vi "Stop_Loop_Case.vi"(6 "Queues":T4, 7 "Timer parameters":refnum<vi>, 8 "Status/Errors in":refnum<vi>, 9 "Control Parameters [] in":T1[](array[typedef]) {"Aux Byte Value" format="%02x"; "Max Real Value" format="%#_6e"; "Min Real Value" format="%#_6e"; "dReal/dByte" format="%#_6e"; "Byte Value" format="%02x"; "Identifier" format="%02x"}, 10 "Main parameters in":T5={"Mode"={"Mode"=enum."Dialog", "Expert?"=FALSE, "Dialog?"=FALSE}, "Stop loop"={"Settings changed?"=FALSE, "Stop?"=refnum}, "Send message"={"Send mode"=enum."Get parameters", "Set parameter list"=0, "Get parameter list"=0, "Reset device"=0, "Length set settings message"=0, "Reset buttons?"=FALSE, "Reset Master?"=enum."General"}, "Write settings"={"Options"=enum."File 1"}, "Settings state"={"MAS locked?"=refnum, "SLV locked?"=refnum}, "Button refs"={"Stop program"=refnum, "Save settings"=refnum, "DAQ mode"=refnum, "Reset settings"=refnum, "Apply settings"=refnum, "Reset MAS"=refnum, "Reset SLV"=refnum, "Local DBase?"=refnum, "Last value DBase"=FALSE, "Database"=refnum, "Calibration"=refnum, "Save settings 2"=refnum}, "Update screen"={"Detector number"=0, "Hardware"=enum."None"}, "Files"={"Path config file"=path "", "Path def. ini file"=path "", "Path ini file 1"=path "", "Path ini file 2"=path "", "Path RBF file"=path ""}, "DB connection"={"connection reference"=refnum, "Connected?"=refnum, "ODBC Name"=""}, "Status_id"=refnum, "Time difference"=refnum, "Satellites"=refnum, "Alignment parameters"=refnum, "Page Statistics 2"=refnum, "Database"=refnum, "Page Statistics"=refnum} {"Update screen"."Detector number" format="%#.0f"; "Send message"."Reset device" format="%x"; "Send message"."Get parameter list" format="%x"; "Send message"."Set parameter list" format="%x"}, 11 "Devices in":T3) -> (1 "Control Parameters [] out":T1[](array[typedef]) {"Aux Byte Value" format="%02x"; "Max Real Value" format="%#_6e"; "Min Real Value" format="%#_6e"; "dReal/dByte" format="%#_6e"; "Byte Value" format="%02x"; "Identifier" format="%02x"}, 2 "Main parameters out":T5={"Mode"={"Mode"=enum."Dialog", "Expert?"=FALSE, "Dialog?"=FALSE}, "Stop loop"={"Settings changed?"=FALSE, "Stop?"=refnum}, "Send message"={"Send mode"=enum."Get parameters", "Set parameter list"=0, "Get parameter list"=0, "Reset device"=0, "Length set settings message"=0, "Reset buttons?"=FALSE, "Reset Master?"=enum."General"}, "Write settings"={"Options"=enum."File 1"}, "Settings state"={"MAS locked?"=refnum, "SLV locked?"=refnum}, "Button refs"={"Stop program"=refnum, "Save settings"=refnum, "DAQ mode"=refnum, "Reset settings"=refnum, "Apply settings"=refnum, "Reset MAS"=refnum, "Reset SLV"=refnum, "Local DBase?"=refnum, "Last value DBase"=FALSE, "Database"=refnum, "Calibration"=refnum, "Save settings 2"=refnum}, "Update screen"={"Detector number"=0, "Hardware"=enum."None"}, "Files"={"Path config file"=path "", "Path def. ini file"=path "", "Path ini file 1"=path "", "Path ini file 2"=path "", "Path RBF file"=path ""}, "DB connection"={"connection reference"=refnum, "Connected?"=refnum, "ODBC Name"=""}, "Status_id"=refnum, "Time difference"=refnum, "Satellites"=refnum, "Alignment parameters"=refnum, "Page Statistics 2"=refnum, "Database"=refnum, "Page Statistics"=refnum} {"Update screen"."Detector number" format="%#.0f"; "Send message"."Reset device" format="%x"; "Send message"."Get parameter list" format="%x"; "Send message"."Set parameter list" format="%x"}, 3 "Devices out":T3)   [LabVIEW 2013]
uses:
  Controls/Main_Parameters.ctl
  Controls/Mode.ctl
  Controls/Stop_Loop.ctl
  Controls/Send_Message.ctl
  Controls/Send_Message_Mode.ctl
  Controls/Master.ctl
  Controls/Write_Settings.ctl
  Controls/Write_Settings_Options.ctl
  Controls/Settings_State.ctl
  Controls/Button_Refs.ctl
  Controls/Update_Screen.ctl
  Controls/Files.ctl
  Controls/DB_Connection.ctl
  database/Connection.llb/Conn ObjectReference.ctl
  Controls/Devices.ctl
  Controls/Control_Parameters.ctl
  Controls/Queues.ctl
  Controls/One_Second.ctl
  Controls/GPS_Timestamp.ctl
panel:
  out "Error":errorcluster
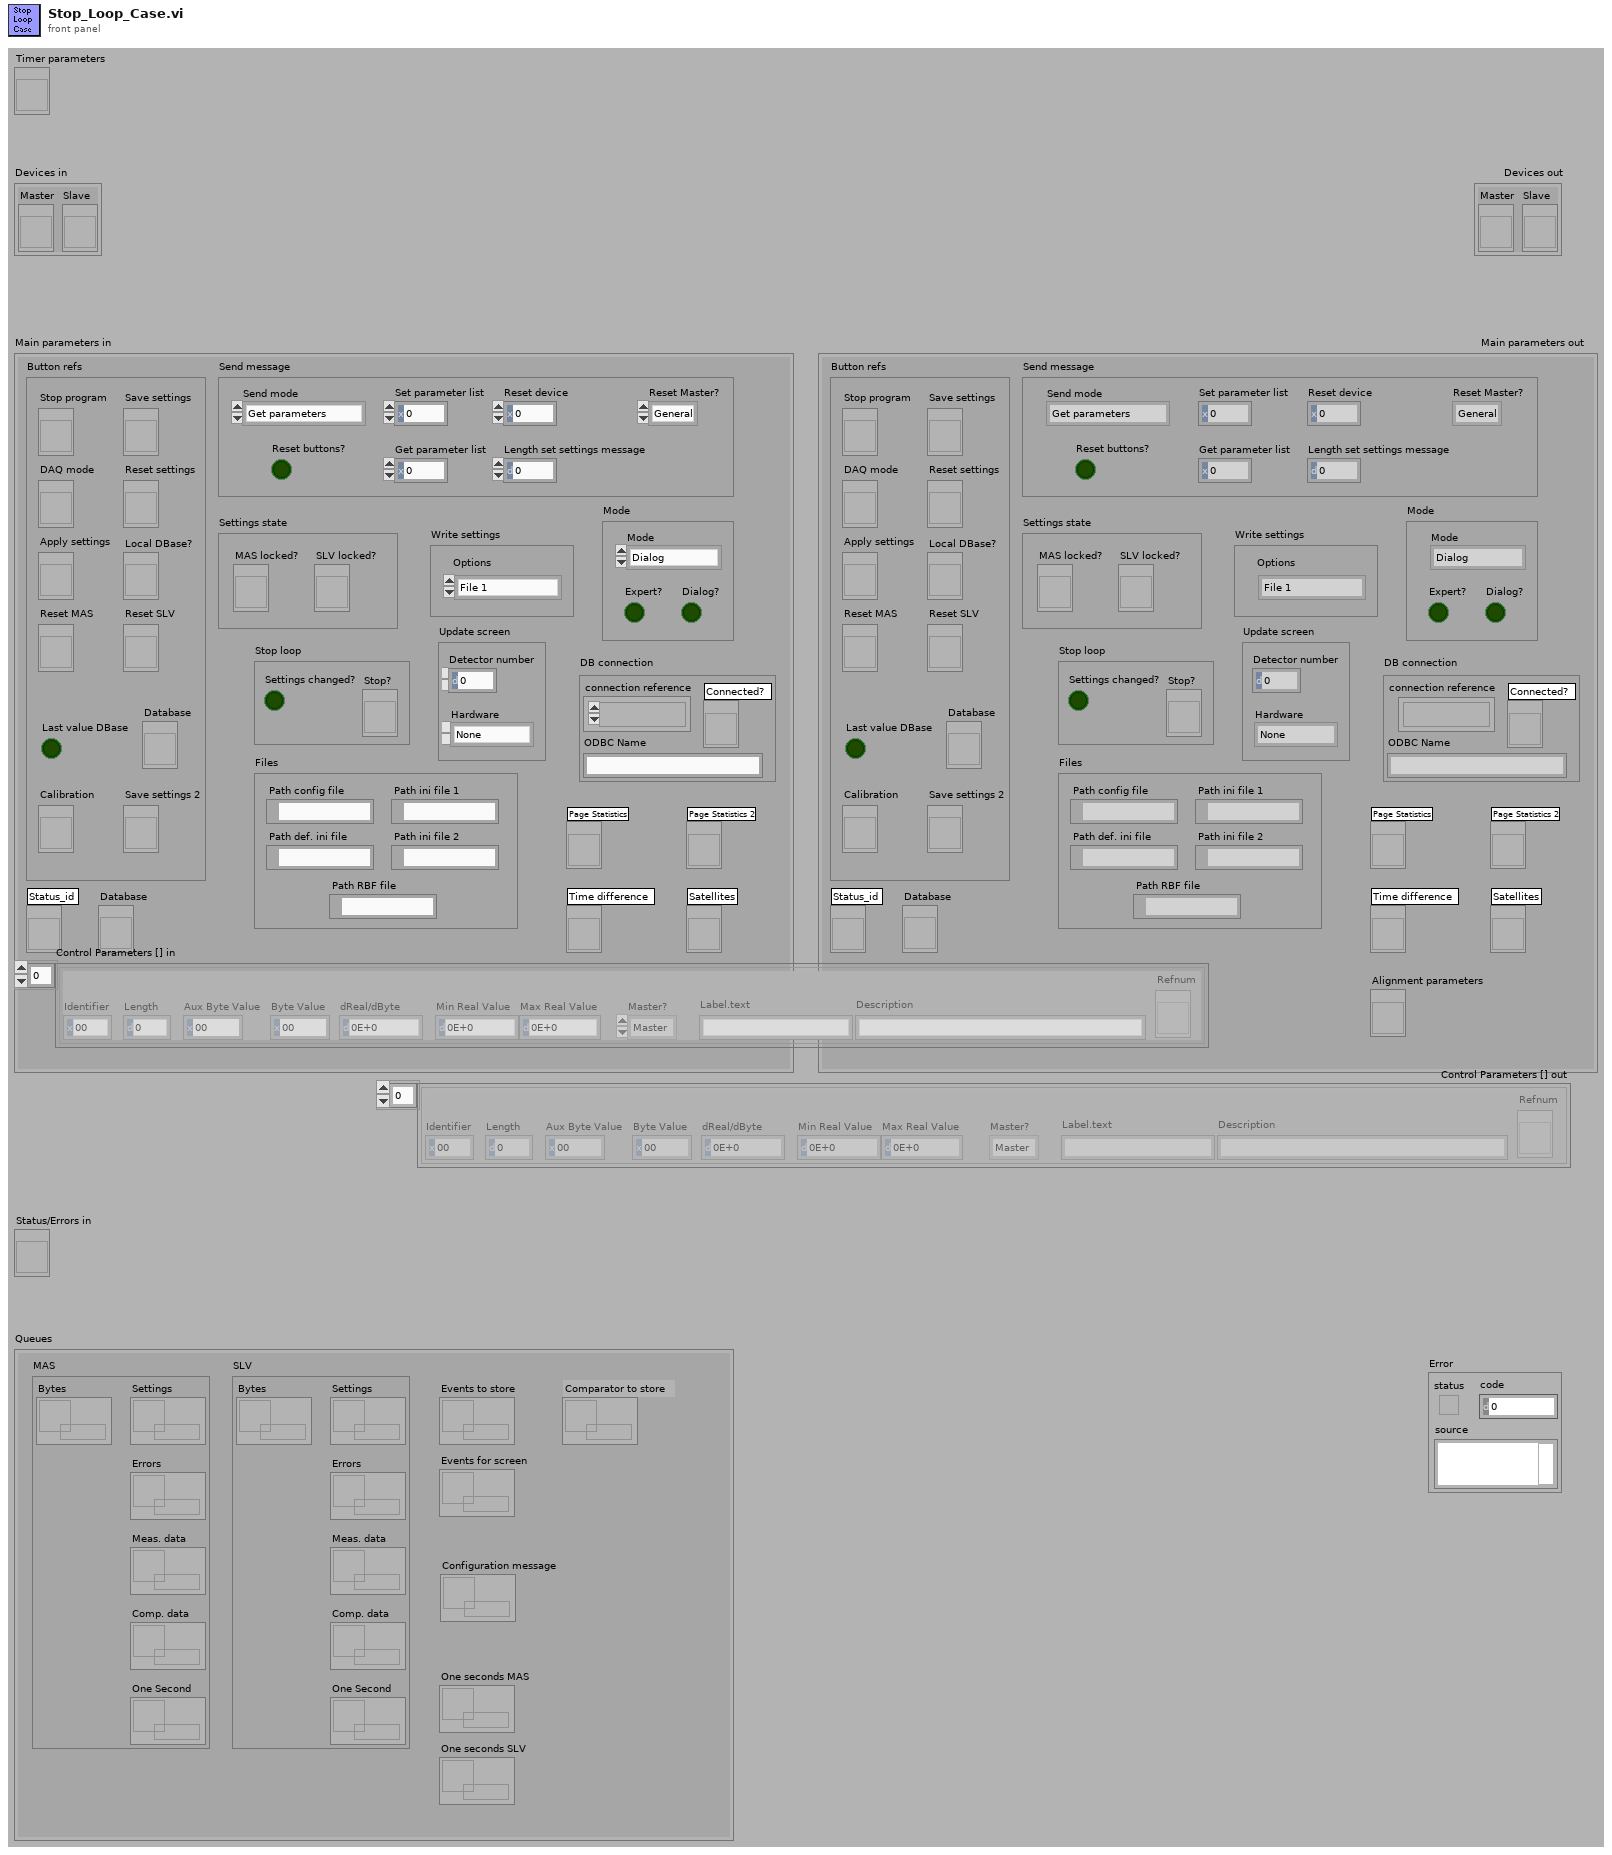
[diagram p1: front panel]
types:
  T1 = typedef "Control_Parameters.ctl" = cluster{"Identifier":u8, "Length":u16, "Byte Value":u32, "dReal/dByte":dbl, "Min Real Value":dbl, "Max Real Value":dbl, "Master?":T2, "Label.text":string, "Description":string, "Refnum":refnum<vi>, "Aux Byte Value":u32}
  T2 = typedef "Master.ctl" = enum16{"Master", "Slave", "General"}
  T3 = typedef "Devices.ctl" = cluster{"Master":refnum<vi>, "Slave":refnum<vi>}
  T4 = typedef "Queues.ctl" = cluster{"MAS":cluster{"Bytes":refnum<queue>, "Settings":refnum<queue>, "Errors":refnum<queue>, "Meas. data":refnum<queue>, "One Second":refnum<queue>, "Comp. data":refnum<queue>}, "SLV":cluster{"Bytes":refnum<queue>, "Settings":refnum<queue>, "Errors":refnum<queue>, "Meas. data":refnum<queue>, "One Second":refnum<queue>, "Comp. data":refnum<queue>}, "Events to store":refnum<queue>, "Events for screen":refnum<queue>, "One seconds MAS":refnum<queue>, "One seconds SLV":refnum<queue>, "Configuration message":refnum<queue>, "Comparator to store":refnum<queue>}
  T5 = typedef "Main_Parameters.ctl" = cluster{"Mode":T6, "Stop loop":T7, "Send message":T8, "Write settings":T10, "Settings state":T12, "Button refs":T13, "Update screen":T14, "Files":T15, "DB connection":T16, "Status_id":refnum<vi>, "Time difference":refnum<vi>, "Satellites":refnum<vi>, "Alignment parameters":refnum<vi>, "Page Statistics 2":refnum<vi>, "Database":refnum<vi>, "Page Statistics":refnum<vi>}
  T6 = typedef "Mode.ctl" = cluster{"Mode":enum8{"Stop", "Dialog", "Hisparc II", "Hisparc II DAQ", "Alignment"}, "Expert?":bool, "Dialog?":bool}
  T7 = typedef "Stop_Loop.ctl" = cluster{"Settings changed?":bool, "Stop?":refnum<vi>}
  T8 = typedef "Send_Message.ctl" = cluster{"Send mode":T9, "Set parameter list":u8, "Get parameter list":u8, "Reset device":u8, "Length set settings message":i32, "Reset buttons?":bool, "Reset Master?":T2}
  T9 = typedef "Send_Message_Mode.ctl" = enum16{"Get parameters", "Set parameters", "From front panel", "From parameters", "Reset device", "Alignment"}
  T10 = typedef "Write_Settings.ctl" = cluster{"Options":T11}
  T11 = typedef "Write_Settings_Options.ctl" = enum16{"File 1", "File 2", "Alignment", "Reset"}
  T12 = typedef "Settings_State.ctl" = cluster{"MAS locked?":refnum<vi>, "SLV locked?":refnum<vi>}
  T13 = typedef "Button_Refs.ctl" = cluster{"Stop program":refnum<vi>, "Save settings":refnum<vi>, "DAQ mode":refnum<vi>, "Reset settings":refnum<vi>, "Apply settings":refnum<vi>, "Reset MAS":refnum<vi>, "Reset SLV":refnum<vi>, "Local DBase?":refnum<vi>, "Last value DBase":bool, "Database":refnum<vi>, "Calibration":refnum<vi>, "Save settings 2":refnum<vi>}
  T14 = typedef "Update_Screen.ctl" = cluster{"Detector number":u16, "Hardware":enum8{"None", "HiSPARC I", "HiSPARC II", "HiSPARC III", "Unknown"}}
  T15 = typedef "Files.ctl" = cluster{"Path config file":path, "Path def. ini file":path, "Path ini file 1":path, "Path ini file 2":path, "Path RBF file":path}
  T16 = typedef "DB_Connection.ctl" = cluster{"connection reference":T17, "Connected?":refnum<vi>, "ODBC Name":string}
  T17 = typedef "Conn ObjectReference.ctl" = refnum<k1>
  T18 = enum16{"Only front panel", "Only buttons", "Both", "Invisible"}
  T19 = typedef "Rendezvous RefNum" = refnum<k1>
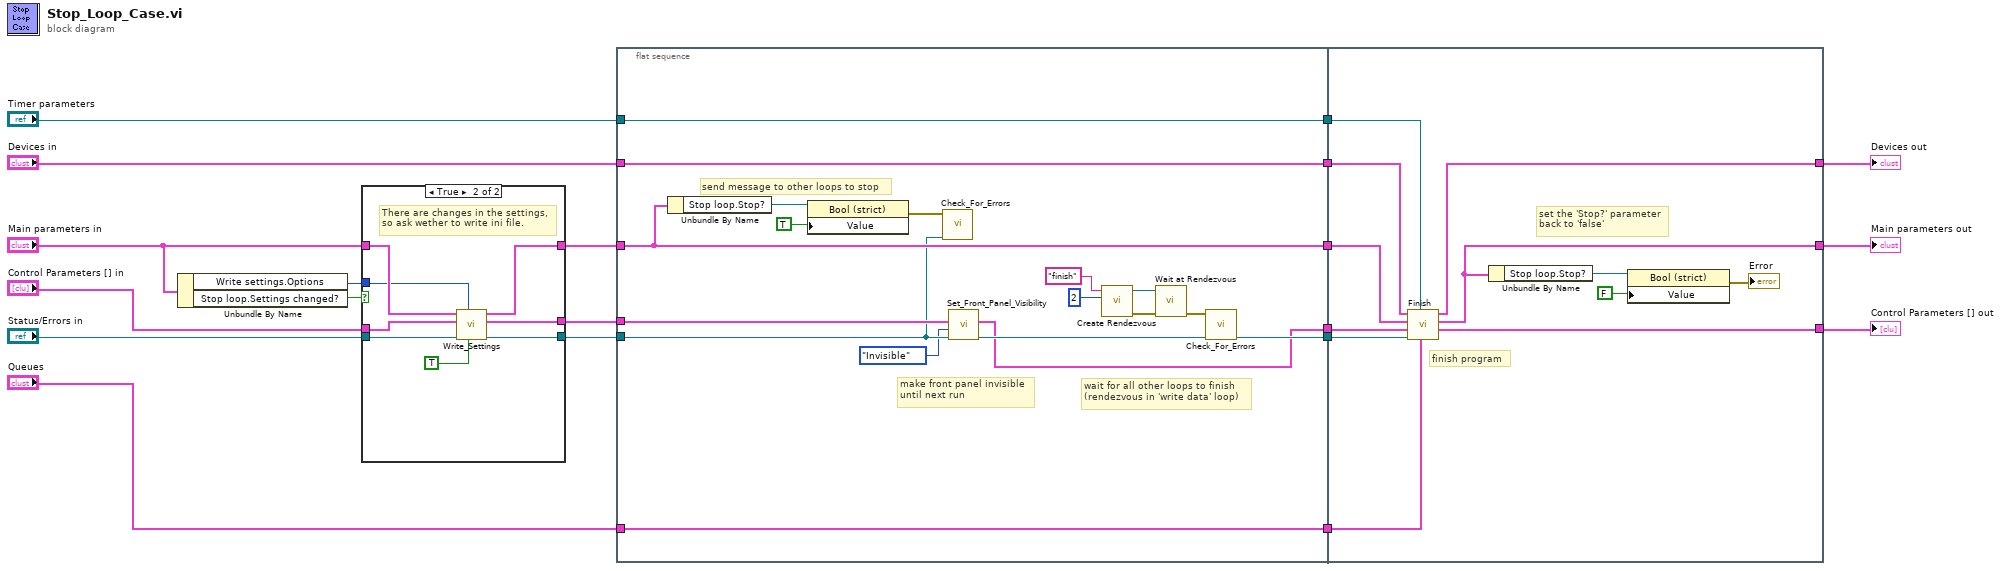
[diagram p0: block diagram]
diagram:
  n1 = Unbundle By Name("Main parameters in") -> ("Write settings.Options"=w16:T11, "Stop loop.Settings changed?"=w20:bool)
  n2 = case shown="True" w20 {
    tunnel: "Status/Errors in" -> [w22 w31]
    tunnel: [w22 w30] -> w8
    tunnel: "Control Parameters [] in" -> [w23 w29]
    tunnel: [w23 w28] -> w6
    tunnel: "Main parameters in" -> [w21 w26]
    tunnel: [w21 w25] -> w7
    tunnel: w16 -> [_ w24]
    frame False {
      # "There are no changes in the\nsettings, so don't write ini file."
    }
    frame True {
      # "There are changes in the settings,\nso ask wether to write ini file."
      n3 = call "Write_Settings.vi"("Dialog? (false)"=TRUE, "Options"=w24, "Status/Errors in"=w31, "Control Parameters [] in"=w29, "Main parameters in"=w26) -> ("Status/Errors out"=w30:refnum<vi>, "Control Parameters [] out"=w28:T1[], "Main parameters out"=w25:T5)  [unwired: 1 in, 3 out]
    }
  }
  n4 = flat-sequence {
    tunnel: w8 -> [w33]
    tunnel: w6 -> [w37]
    tunnel: "Devices in" -> [w48]
    tunnel: "Timer parameters" -> [w49]
    tunnel: w7 -> [w43]
    tunnel: [w43] -> w15
    tunnel: [w49] -> w14
    tunnel: [w48] -> w13
    tunnel: [w36] -> w12
    tunnel: [w40] -> w11
    tunnel: [w39] -> w10
    tunnel: "Queues" -> [w39]
    tunnel: [w51] -> w3
    tunnel: [w55] -> w4
    tunnel: [w54] -> w2
    tunnel: w15 -> [w59]
    tunnel: w14 -> [w57]
    tunnel: w13 -> [w58]
    tunnel: w12 -> [w61]
    tunnel: w11 -> [w60]
    tunnel: w10 -> [w56]
    frame #0 {
      # "make front panel invisible\nuntil next run"
      # "send message to other loops to stop"
      # "wait for all other loops to finish\n(rendezvous in 'write data' loop)"
      n5 = Unbundle By Name(w43) -> ("Stop loop.Stop?"=w47:refnum<vi>)
      n6 = property class="Bool (strict)"(reference=w47, "Value"=TRUE) -> (error out=w34:errorcluster)  [unwired: 1 in, 1 out]
      n7 = call "Check_For_Errors.vi"("Status/Errors in"=w33, "error in"=w34) -> ()  [unwired: 10 out]
      n8 = call "Set_Front_Panel_Visibility.vi"("Status/Errors in"=w33, "Visibility"=T18."Invisible", "Control Parameters [] in"=w37) -> ("Status/Errors out"=w38:refnum<vi>, "Control Parameters [] out"=w36:T1[])  [unwired: 1 in, 6 out]
      n9 = call <vilib>:"Create Rendezvous.vi"("size (2)"=2, "name (unnamed)"="finish") -> ("error out"=w44:errorcluster, "rendezvous"=w45:T19)  [unwired: 1 in, 3 out]
      n10 = call <vilib>:"Wait at Rendezvous.vi"("error in (no error)"=w44, "rendezvous"=w45) -> ("error out"=w35:errorcluster)  [unwired: 1 in, 4 out]
      n11 = call "Check_For_Errors.vi"("Status/Errors in"=w38, "error in"=w35) -> ("Status/Errors out"=w40:refnum<vi>)  [unwired: 9 out]
    }
    frame #1 {
      # "finish program"
      # "set the 'Stop?' parameter\nback to 'false'"
      n12 = call "Finish.vi"("Queues"=w56, "Timer parameters"=w57, "Status/Errors in"=w60, "Control Parameters [] in"=w61, "Main parameters in"=w59, "Devices in"=w58) -> ("Control Parameters [] out"=w55:T1[], "Main parameters out"=w51:T5, "Devices out"=w54:T3)  [unwired: 1 in, 2 out]
      n13 = Unbundle By Name(w51) -> ("Stop loop.Stop?"=w53:refnum<vi>)
      n14 = property class="Bool (strict)"(reference=w53, "Value"=FALSE) -> (error out=→"Error":errorcluster)  [unwired: 1 in, 1 out]
    }
  }
  "Main parameters out" <- w3
  "Devices out" <- w2
  "Control Parameters [] out" <- w4
